vi "find_label_indicies.vi"(10 "Array":T2[](array[typedef])=[{"Label Array"=["MixingTeedP", "PGinlet-MixingTeePressure", "PGinlet-MixingTeeTemperature"]}, {"Label Array"=["AtmosphericPressure"]}, {"Label Array"=["LiquidTankPressure", "LiquidTankTemperature", "SeparatorPressure", "SeparatorTemperature", "LiquidInletPressure", "LiquidInletTemperature", "VaporTankPressure", "VaporTankTemperature", "VaporInletPressure", "VaporInletTemperature", "TSWindow1AbsolutePressure", "TSWindow1Temperature", "UpperDevSectionPressure", "UpperDevSectionTemperature", "LowerDevSectionPressure", "UpperDevSectionTemperature"]}, {"Label Array"=["VaporLineDensity", "LiquidLineDensity"]}, {"Label Array"=["VaporInletPressure", "LiquidMassFlow", "VaporMassFlow", "LiquidInletTemperature", "SeparatorTemperature"]}, {"Label Array"=["PGAbsolutePressure", "PGVaporTemperature", "PGLiquidTemperature", "TSWindow1Temperature", "TSWindow7Temperature", "TSWindow1AbsolutePressure", "TSWindow7AbsolutePressure", "Window1to4dP", "Window1to7dP", "Window1to7FastdP", "PGPitotdP", "VaporLinePitotdP"]}, {"Label Array"=["MainDiode", "ControlDiode", "TSExteriorTemperature", "TSWindow1AbsolutePressure"]}], 11 "haystack":T3[](array[typedef])) -> (2 "Indicies":T1[](array[typedef]), 3 "Needles Out":T3[][](array[typedef]))   [LabVIEW 2017]
uses:
  Box/Annular Flow/Jason/LabVIEW 2017/Input Channel Lists/analog_data.ctl
  label_array_cluster.ctl
  index_array_cluster.ctl
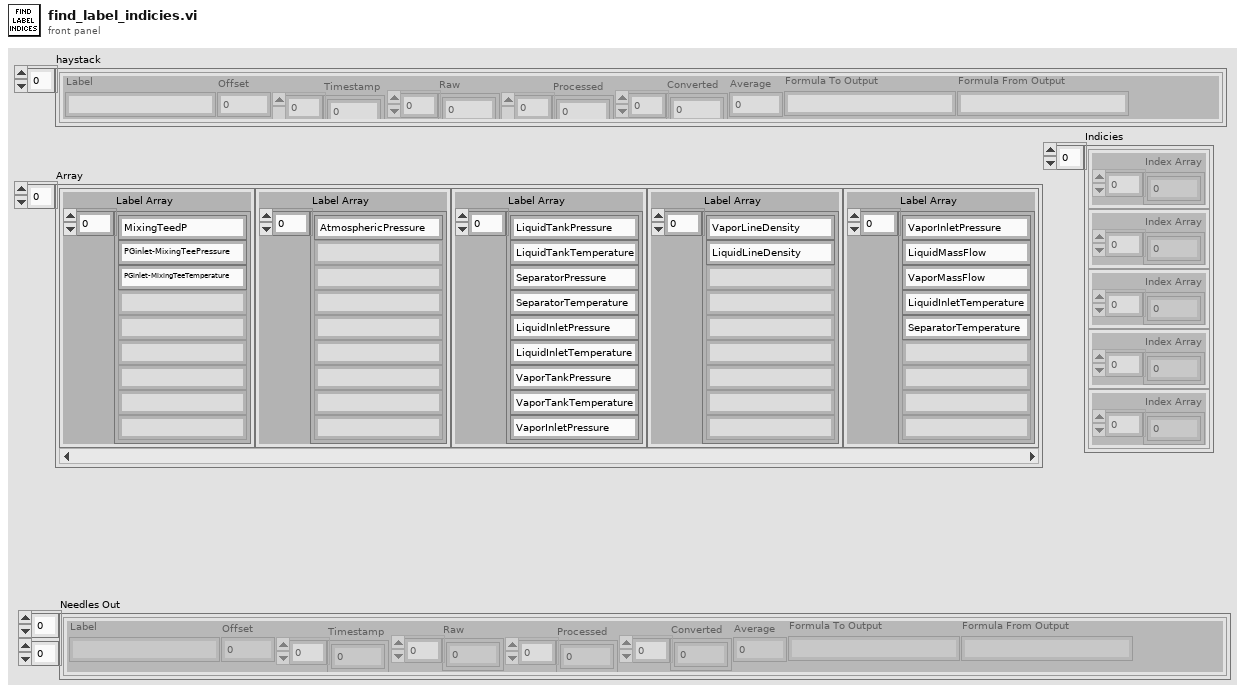
[diagram p1: front panel]
types:
  T1 = typedef "index_array_cluster.ctl" = cluster{"Index Array":i32[]}
  T2 = typedef "label_array_cluster.ctl" = cluster{"Label Array":string[]}
  T3 = typedef "analog_data.ctl" = cluster{"Label":string, "Offset":dbl, "Timestamp":dbl[], "Raw":dbl[], "Processed":dbl[], "Converted":dbl[], "Average":dbl, "Formula To Output":string, "Formula From Output":string}
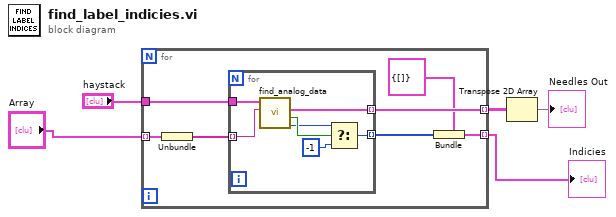
[diagram p0: block diagram]
diagram:
  n1 = for {
    tunnel: "Array" -> [w10] mode=indexing
    tunnel: "haystack" -> [w12]
    tunnel: [w7] -> w1 mode=indexing
    tunnel: [w11] -> w4 mode=indexing
    n2 = Unbundle(w10) -> ("Label Array"=w9:string[])
    n3 = for {
      tunnel: w9 -> [w18] mode=indexing
      tunnel: w12 -> [w19]
      tunnel: [w14] -> w8 mode=indexing
      tunnel: [w13] -> w11 mode=indexing
      n4 = call "find_analog_data.vi"("Needle"=w18, "Haystack"=w19) -> ("Index"=w16:i32, "Found?"=w17:bool, "Needle Out"=w13:T3)  [unwired: 7 in]
      n5 = Select(t=w16, s=w17, f=-1) -> (s? t:f=w14:i32)
    }
    n6 = Bundle(cluster=T1 {"Index Array"=[]} ("Refnum Array Cluster"), "Index Array"=w8) -> (w7:T1)
  }
  "Indicies" <- w1
  n7 = Transpose 2D Array(2D array=w4) -> (transposed array=→"Needles Out":T3[][])
